vi "Stop Trigger Logical Channel.vi"(8 "error in (no error)":errorcluster, 10 "12 Digitals inputs state":T1[](array[typedef]) items=["Off", "On", "Ignore"], 11 "VISA resource name":refnum<visa-resource-name>) -> (0 "error out":errorcluster, 3 "VISA resource name out":refnum<visa-resource-name>)   [LabVIEW 2017, in "Sefram DAS220.lvlib"]
doc: "Stop recording on an event on logical channels.\nFor example : to start if DI0 is on high state, the mask should be setup as DI0 is \"On\" and others in \"Ignore\" state."
uses:
  <instrlib>/Sefram DAS220/Sefram DAS220.lvlib
  <instrlib>/Sefram DAS220/Public/Configure/Triggers-Alarms/Low-level/Trigger Types/Logical TriState.ctl
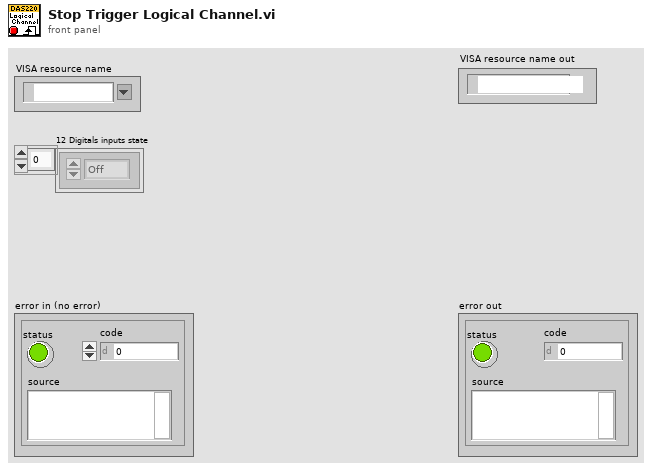
[diagram p1: front panel]
types:
  T1 = typedef "Sefram DAS220.lvlib/Logical TriState.ctl" = u16
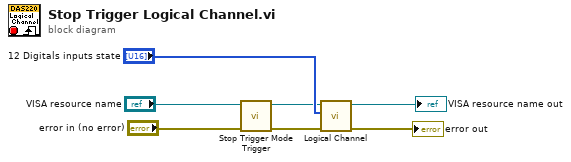
[diagram p0: block diagram]
diagram:
  n1 = call <instrlib>:"Stop Trigger Mode Trigger.vi"("error in (no error)"="error in (no error)", "VISA resource name"="VISA resource name") -> ("error out"=w1:errorcluster, "VISA resource name out"=w2:refnum<visa-resource-name>)  [unwired: 8 in]
  n2 = call <instrlib>:"Logical Channel.vi"("error in (no error)"=w1, "12 Logicals inputs state"="12 Digitals inputs state", "VISA resource name"=w2) -> ("error out"=→"error out":errorcluster, "VISA resource name out"=→"VISA resource name out":refnum<visa-resource-name>)  [unwired: 7 in]
